vi "Check Type.vi"(8 "error in":errorcluster, 11 "Value in":variant) -> (0 "error out":errorcluster, 2 "Type":enum16{"Value", "Future", "Rejected"}(ring), 3 "Value out":variant)   [LabVIEW 2017, in "Promise Future.lvlib" / "Future.lvclass"]
uses:
  Future.lvclass
  Rejected Future/Rejected Future.lvclass
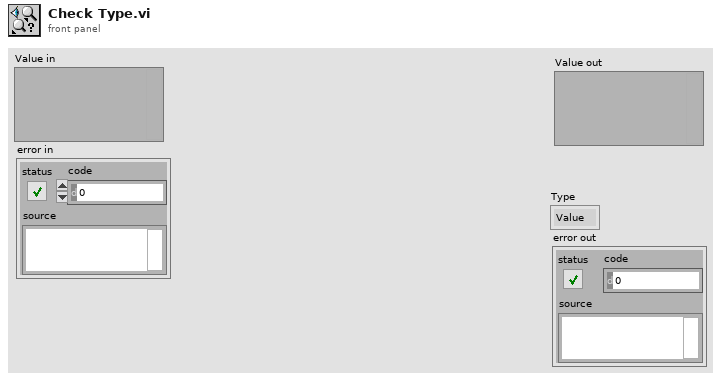
[diagram p1: front panel]
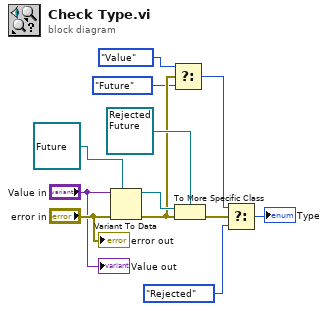
[diagram p0: block diagram]
diagram:
  n1 = Variant To Data(error in="error in", type=refnum<class "Future.lvclass"> refnum ("Future in"), Variant="Value in") -> (data=w10:refnum<class "Future.lvclass">, error out=w7:errorcluster)
  n2 = Select(t=enum16{"Value", "Future", "Rejected"}."Value", s=w7, f=enum16{"Value", "Future", "Rejected"}."Future") -> (s? t:f=w4:enum16{"Value", "Future", "Rejected"})
  n3 = To More Specific Class(target class=refnum<class "Rejected Future.lvclass"> refnum ("Promise Future.lvlib:Rejected Future.lvclass"), reference=w10, error in=w7) -> (error out=w9:errorcluster)  [unwired: 1 out]
  n4 = Select(t=w4, s=w9, f=enum16{"Value", "Future", "Rejected"}."Rejected") -> (s? t:f=→"Type":enum16{"Value", "Future", "Rejected"})
  "error out" <- "error in"
  "Value out" <- "Value in"
